vi "SL TAGS Get Server Tag Update Count.vi"(8 "error in (no error)":errorcluster, 11 "EEISysLink in":refnum<class "EEISysLink.lvclass">) -> (0 "error out":errorcluster, 2 "Tag Server Updates":i32, 3 "EEISysLink out":refnum<class "EEISysLink.lvclass">)   [LabVIEW 2017, in "EEISysLink.lvclass"]
doc: "Get the number of updates from the SystemLink server. This currently comes from the first tag that returns the aggregate count. \n\nJames Tillett P.E.\nEndeavor Engineering Inc.\nwww.endeavoreng.com"
uses:
  EEISysLink.lvclass
  EEISysLink.lvclass/EEISysLink.ctl
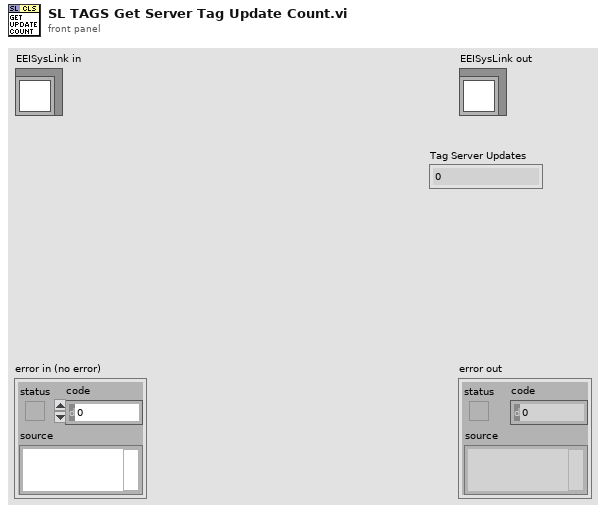
[diagram p1: front panel]
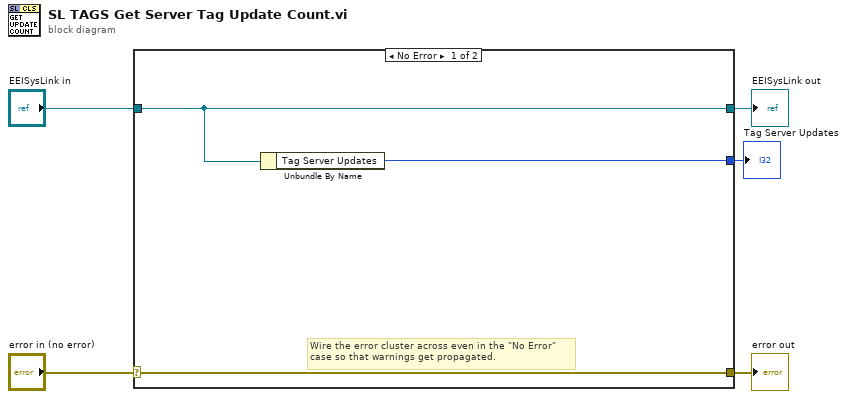
[diagram p0: block diagram]
diagram:
  n1 = case shown="No Error" "error in (no error)" {
    selector: "error in (no error)" -> [w8 w10]
    tunnel: [w8 w10] -> w4
    tunnel: [w7 w9] -> w2
    tunnel: "EEISysLink in" -> [w7 w9]
    tunnel: [w6 _] -> w1
    frame No Error {
      # "Wire the error cluster across even in the \"No Error\"\ncase so that warnings get propagated."
      n2 = Unbundle By Name(w7) -> ("Tag Server Updates"=w6:i32)
    }
    frame Error {
    }
  }
  "error out" <- w4
  "EEISysLink out" <- w2
  "Tag Server Updates" <- w1
